vi "Read.vi"(8 "error in (no error)":errorcluster, 11 "HAL.Serial in":refnum<class "HAL.Serial.lvclass">) -> (0 "error out":errorcluster, 2 "response":string, 3 "HAL.Serial out":refnum<class "HAL.Serial.lvclass">)   [LabVIEW 2019, in "HAL.Serial.lvclass"]
doc: "Override to <b>close</b> the connection to your hardware"
uses:
  HAL.Serial.lvclass
  HAL.Serial.lvclass/HAL.Serial.ctl
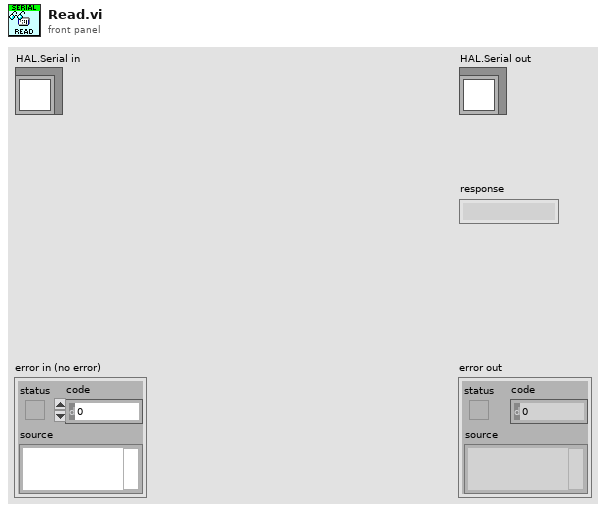
[diagram p1: front panel]
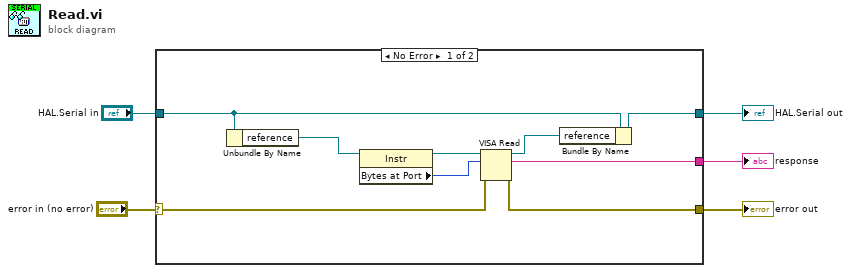
[diagram p0: block diagram]
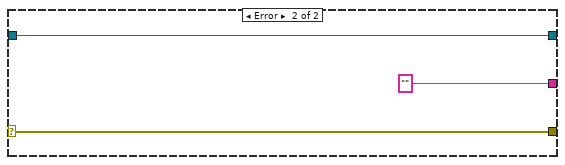
[diagram p2: hidden frame]
diagram:
  n1 = case shown="No Error" "error in (no error)" {
    selector: "error in (no error)" -> [w14 w17]
    tunnel: [w13 w17] -> w3
    tunnel: "HAL.Serial in" -> [w12 w16]
    tunnel: [w11 w16] -> w2
    tunnel: [w9 "" ("read buffer")] -> w1
    frame No Error {
      n2 = Unbundle By Name(w12) -> ("reference"=w7:refnum<visa-resource-name>)
      n3 = property class="Instr"(reference=w7) -> (reference out=w6:refnum<visa-resource-name>, "Bytes at Port"=w8:u32)  [unwired: 1 in, 1 out]
      n4 = VISA Read(VISA resource name=w6, byte count=w8, error in (no error)=w14) -> (VISA resource name out=w10:refnum<visa-resource-name>, read buffer=w9:string, error out=w13:errorcluster)  [unwired: 1 out]
      n5 = Bundle By Name(cluster=w12, "reference"=w10) -> (w11:refnum<class "HAL.Serial.lvclass">)
    }
    frame Error {
    }
  }
  "error out" <- w3
  "HAL.Serial out" <- w2
  "response" <- w1
